vi "Other Output Item Resize.vi"(8 "error in (no error)":errorcluster, 9 "NewBnds":T2, 10 "Other UI Elements":T1) -> (0 "error out":errorcluster)   [LabVIEW 2015, in "OutputUI.lvclass"]
uses:
  OutputUI.lvclass
  <vilib>/Utility/miscctls.llb/LVRectTypeDef.ctl
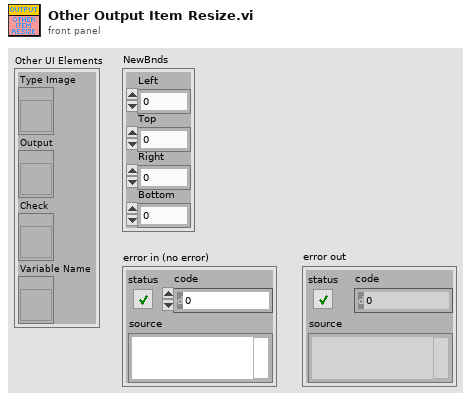
[diagram p1: front panel]
types:
  T1 = cluster{"Type Image":refnum<vi>, "Output":refnum<vi>, "Check":refnum<vi>, "Variable Name":refnum<vi>}
  T2 = typedef "LVRectTypeDef.ctl" = cluster{"Left":i16, "Top":i16, "Right":i16, "Bottom":i16}
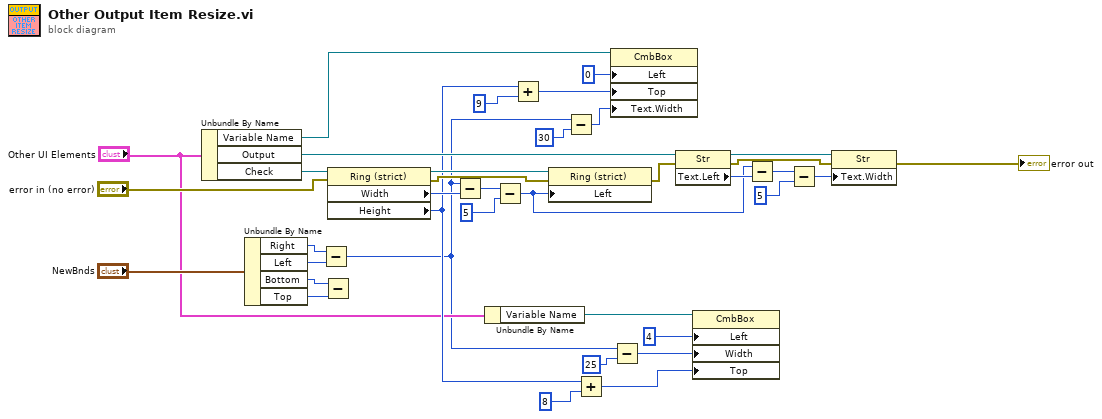
[diagram p0: block diagram]
diagram:
  n1 = Unbundle By Name("Other UI Elements") -> ("Variable Name"=w15:refnum<vi>, "Output"=w29:refnum<vi>, "Check"=w37:refnum<vi>)
  n2 = Unbundle By Name("NewBnds") -> ("Right"=w34:i16, "Left"=w35:i16, "Bottom"=w33:i16, "Top"=w32:i16)
  n3 = Subtract(x=w34, y=w35) -> (x-y=w1:i16)
  n4 = Subtract(x=w33, y=w32) -> ()  [unwired: 1 out]
  n5 = property class="Ring (strict)"(reference=w37, error in="error in (no error)") -> (reference out=w31:refnum<vi>, error out=w18:errorcluster, "Width"=w30:u32, "Height"=w11:u32)
  n6 = Subtract(x=w1, y=w30) -> (x-y=w26:u32)
  n7 = Unbundle By Name("Other UI Elements") -> ("Variable Name"=w7:refnum<vi>)
  n8 = Subtract(x=w26, y=5) -> (x-y=w24:u32)
  n9 = Add(x=w11, y=9) -> (x+y=w12:u32)
  n10 = property class="Ring (strict)"(reference=w31, error in=w18, "Left"=w24) -> (error out=w17:errorcluster)  [unwired: 1 out]
  n11 = Subtract(x=w1, y=30) -> (x-y=w10:i32)
  n12 = Add(x=w11, y=8) -> (x+y=w3:u32)
  n13 = property class="CmbBox"(reference=w15, "Left"=0 ("Position:Left"), "Top"=w12, "Text.Width"=w10) -> ()  [unwired: 1 in, 2 out]
  n14 = Subtract(x=w1, y=u32 25) -> (x-y=w4:u32)
  n15 = property class="Str"(reference=w29, error in=w17) -> (reference out=w28:refnum<vi>, error out=w16:errorcluster, "Text.Left"=w27:i32)
  n16 = property class="CmbBox"(reference=w7, "Left"=4 ("Position:Left"), "Width"=w4, "Top"=w3) -> ()  [unwired: 1 in, 2 out]
  n17 = Subtract(x=w24, y=w27) -> (x-y=w23:u32)
  n18 = Subtract(x=w23, y=u32 5) -> (x-y=w22:u32)
  n19 = property class="Str"(reference=w28, error in=w16, "Text.Width"=w22) -> (error out=→"error out":errorcluster)  [unwired: 1 out]
